vi "x502_stop.vi"(2 "error in (no error)":errorcluster, 3 "x502 in":refnum<k24>) -> (0 "error out":errorcluster, 1 "x502 out":refnum<k24>)   [LabVIEW 2010]
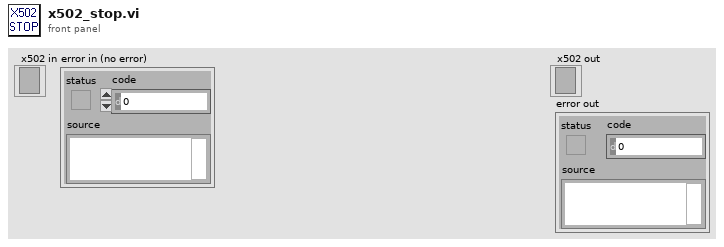
[diagram p1: front panel]
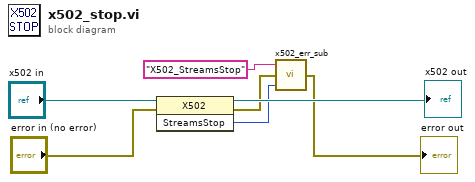
[diagram p0: block diagram]
diagram:
  n1 = invoke class="X502" method="StreamsStop"(reference="x502 in", error in="error in (no error)") -> (reference out=→"x502 out":refnum<k24>, error out=w6:errorcluster, "StreamsStop"=w4:i32)  [unwired: 1 in]
  n2 = call "x502_err_sub.vi"("Error code"=w4, "error in (no error)"=w6, "Error descr"="X502_StreamsStop") -> ("error out"=→"error out":errorcluster)
